vi "Front Panel Info.vi"(4 "VI Reference":refnum<vi>) -> (0 "Width":u32, 1 "Height":u32, 2 "Front Panel Refernce":refnum<vi>)   [LabVIEW 2013]
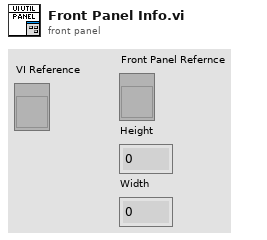
[diagram p1: front panel]
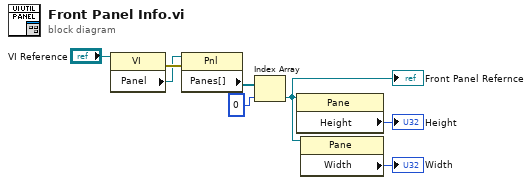
[diagram p0: block diagram]
diagram:
  n1 = property class="VI"(reference="VI Reference") -> (error out=w8:errorcluster, "Panel"=w3:refnum<vi>)  [unwired: 1 in, 1 out]
  n2 = property class="Pnl"(reference=w3, error in=w8) -> ("Panes[]"=w7:refnum<vi>[])  [unwired: 2 out]
  n3 = Index Array(array=w7, index=0) -> (element=w5:refnum<vi>)
  "Front Panel Refernce" <- w5
  n4 = property class="Pane"(reference=w5) -> ("Height"=→"Height":u32)  [unwired: 1 in, 2 out]
  n5 = property class="Pane"(reference=w5) -> ("Width"=→"Width":u32)  [unwired: 1 in, 2 out]
